vi "Read Ports_modified.vi"(0 "Refnum in":refnum<k20>, 2 "timeout (ms)":i32=5000, 5 "2 Ports":bool, 9 "number of elements":u64, 11 "error in":errorcluster) -> (4 "Refnum out":refnum<k20>, 6 "Read Region References":refnum<data-value>[](array[refnum]), 8 "Errors":u32[](array[numeric]), 10 "Elements Remaining":u32, 14 "Data Valid":bool, 15 "error out":errorcluster)   [LabVIEW 2016, in "Aurora Stream (NI 6592R) (Host).lvlib"]
doc: "This VI wraps and calls the appropriate FIFO read node to access the FIFO corresponding to the input <b>port</b>\n\n<B>Input Parameters</B>\n\n<B>Refnum in</B> Receives a reference to the FPGA from the previous VI.\n\n<B>timeout (ms)</B> The timeout to pass to the FIFO read node\n\n<B>port</B> Selects which physical port to read from.\n\n<B>number of elements</B> Specifies the number of FIFO elements to read during this call.\n\n<B>error in</B> describes error conditions that occur before this node runs. This input provides standard error in functionality.\n\n<B>Output Parameters</B>\n\n<B>Refnum out</B> passes a reference to the FPGA to the next VI.\n\n<B>Receive Waveform</B> The data read from the device will be written to this output\n\n<B>Waveform Size</B> Indicates the number of samples in the output waveform\n\n<B>Elements Remaining</B> Indicates the number of samples presently waiting in the FIFO after the read.\n\n<B>error out</B> contains error information. This output provides standard error out functionality."
uses:
  Aurora Stream (NI 6592R) (Host).lvlib
  Base Bitfile Reference.ctl
  <vilib>/rvi/errors/niLvFpgaAdjustHostInterfaceError.vi
  <vilib>/Utility/error.llb/Error Cluster From Error Code.vi
  <vilib>/rvi/interface/nirviReadWriteControl/nirviReadWriteControl.xnode
  <vilib>/rvi/interface/nirviMethod/nirviMethod.xnode
  <vilib>/rvi/errors/niLvFpgaMergeErrorWithErrorCode.vi
  NiFpgaLv.dll
  <vilib>/rvi/interface/Simulation/niFpgaSimulationCallBeginRW.vi
  <vilib>/FPGAPlugInAG/Dynamic/niLvFpga_AcquireReadRegionFifo_Dynamic.vi
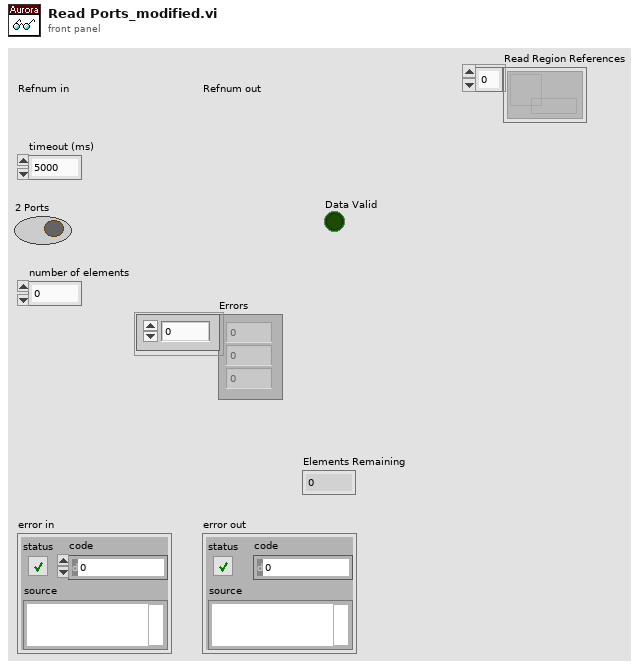
[diagram p1: front panel]
types:
  T1 = typedef "Aurora Stream (NI 6592R) (Host).lvlib/Base Bitfile Reference.ctl" = refnum<k20>
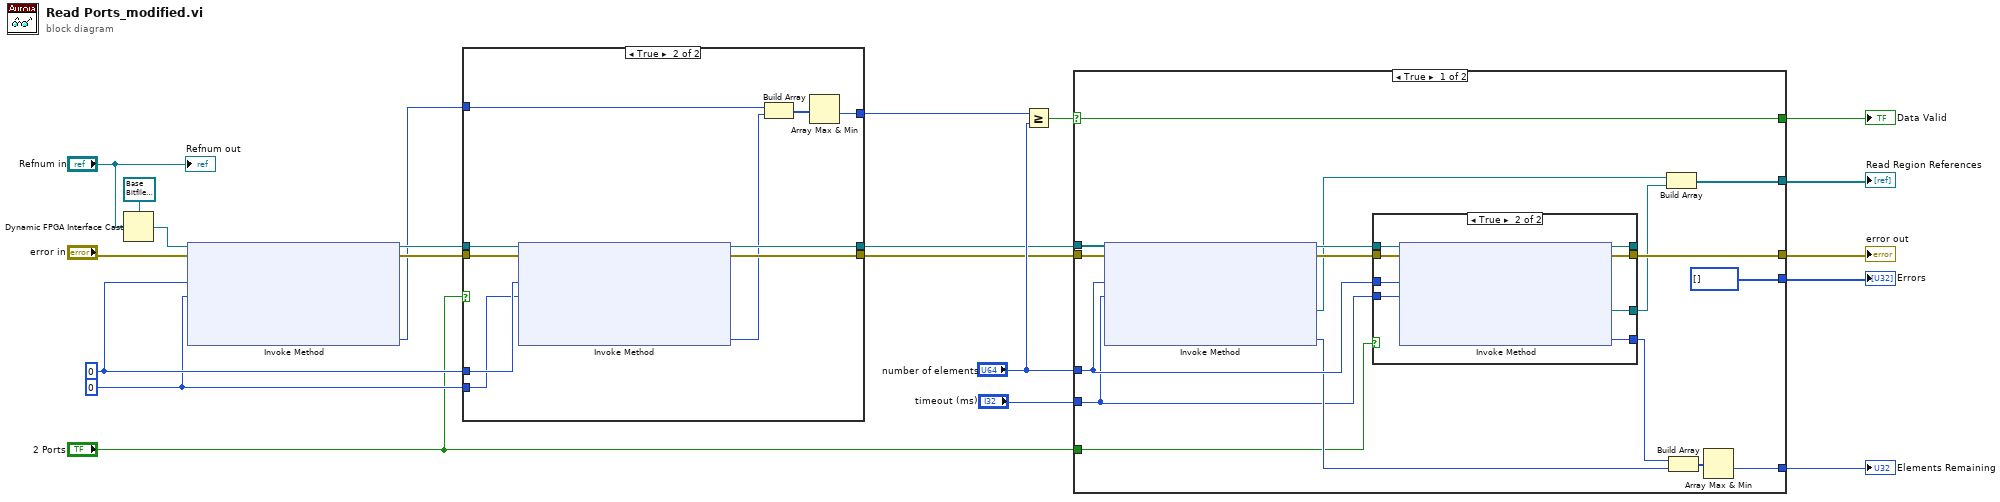
[diagram p0: block diagram]
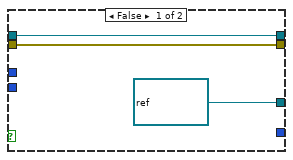
[diagram p3: hidden frame]
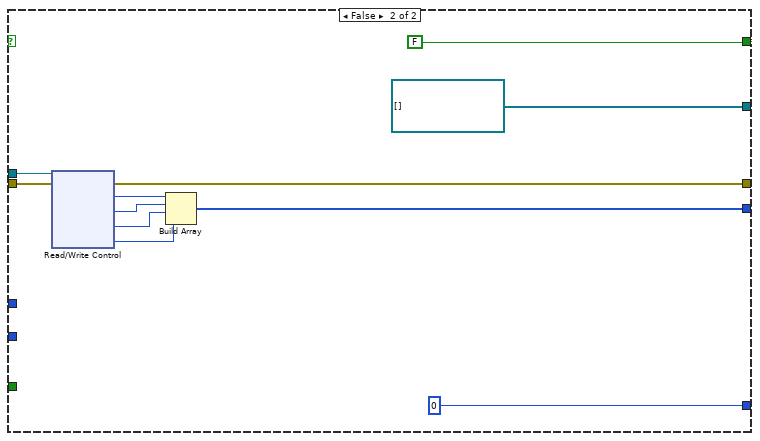
[diagram p4: hidden frame]
diagram:
  w6 = 0 ("Timeout (ms)")
  w7 = u32 0 ("Number of Elements")
  n1 = Dynamic FPGA Interface Cast(Session In=T1 refnum ("Aurora Sample Project"), Type="Refnum in") -> (Session Out=w13:T1)
  n2 = xnode "Invoke Method"("FPGA VI Reference In"=w13, "error in"="error in", "Number of Elements"=w7, "Timeout (ms)"=w6) -> ("FPGA VI Reference Out"=w11:T1, "error out"=w10:errorcluster, "Elements Remaining"=w2:u32)  [unwired: 2 out]
  n3 = case shown="True" "2 Ports" {
    tunnel: w11 -> [w24 w34]
    tunnel: w10 -> [w23 w33]
    tunnel: [w23 w32] -> w9
    tunnel: [w24 w31] -> w8
    tunnel: w7 -> [_ w30]
    tunnel: w6 -> [_ w29]
    tunnel: w2 -> [w22 w28]
    tunnel: [w22 w26] -> w1
    frame False {
    }
    frame True {
      n4 = xnode "Invoke Method"("FPGA VI Reference In"=w34, "error in"=w33, "Number of Elements"=w30, "Timeout (ms)"=w29) -> ("FPGA VI Reference Out"=w31:T1, "error out"=w32:errorcluster, "Elements Remaining"=w27:u32)  [unwired: 2 out]
      n5 = Build Array(w28, w27) -> (w25:u32[])
      n6 = Array Max & Min(array=w25) -> (min value=w26:u32)  [unwired: 3 out]
    }
  }
  n7 = Greater Or Equal?(x=w1, y="number of elements") -> (x >= y?=w17:bool)
  n8 = case shown="True" w17 {
    selector: w17 -> [w42 _]
    tunnel: [w47 w71] -> w21
    tunnel: "timeout (ms)" -> [w39 _]
    tunnel: w9 -> [w51 w72]
    tunnel: "number of elements" -> [w48 _]
    tunnel: "2 Ports" -> [w35 _]
    tunnel: [w45 u32 0] -> w15
    tunnel: [w36 refnum<data-value>[] []] -> w4
    tunnel: [u32[] [] w66] -> w14
    tunnel: w8 -> [w43 w65]
    tunnel: [w42 FALSE] -> w5
    frame True {
      n9 = xnode "Invoke Method"("FPGA VI Reference In"=w43, "error in"=w51, "Number of Elements"=w48, "Timeout (ms)"=w39) -> ("FPGA VI Reference Out"=w49:T1, "error out"=w50:errorcluster, "Read Region Reference"=w37:refnum<data-value>, "Elements Remaining"=w40:u32)  [unwired: 1 out]
      n10 = case shown="True" w35 {
        tunnel: w50 -> [w53 w62]
        tunnel: w49 -> [w54 w61]
        tunnel: [w53 w60] -> w47
        tunnel: [w54 w59] -> _
        tunnel: w48 -> [_ w58]
        tunnel: [_ w57] -> w41
        tunnel: w39 -> [_ w56]
        tunnel: [refnum<data-value> refnum ("Read Region Reference") w55] -> w38
        frame False {
        }
        frame True {
          n11 = xnode "Invoke Method"("FPGA VI Reference In"=w61, "error in"=w62, "Number of Elements"=w58, "Timeout (ms)"=w56) -> ("FPGA VI Reference Out"=w59:T1, "error out"=w60:errorcluster, "Read Region Reference"=w55:refnum<data-value>, "Elements Remaining"=w57:u32)  [unwired: 1 out]
        }
      }
      n12 = Build Array(w37, w38) -> (w36:refnum<data-value>[])
      n13 = Build Array(w41, w40) -> (w46:u32[])
      n14 = Array Max & Min(array=w46) -> (min value=w45:u32)  [unwired: 3 out]
    }
    frame False {
      n15 = xnode "Read/Write Control"("FPGA VI Reference In"=w65, "error in"=w72) -> ("error out"=w71:errorcluster, "Er.Port 0"=w70:u32, "Er.Port 1"=w69:u32, "Er.Port 2"=w68:u32, "Er.Port 3"=w67:u32)  [unwired: 1 out]
      n16 = Build Array(w70, w69, w68, w67) -> (w66:u32[])
    }
  }
  "error out" <- w21
  "Elements Remaining" <- w15
  "Errors" <- w14
  "Data Valid" <- w5
  "Read Region References" <- w4
  "Refnum out" <- "Refnum in"
